vi "Video.vi"(8 "error in (no error)":errorcluster, 9 "title":string, 10 "id":string, 11 "Video in":refnum<class "Video.lvclass">) -> (0 "error out":errorcluster, 3 "Video out":refnum<class "Video.lvclass">)   [LabVIEW 2017, in "Video.lvclass"]
uses:
  Video.lvclass
  Video.lvclass/Video.ctl
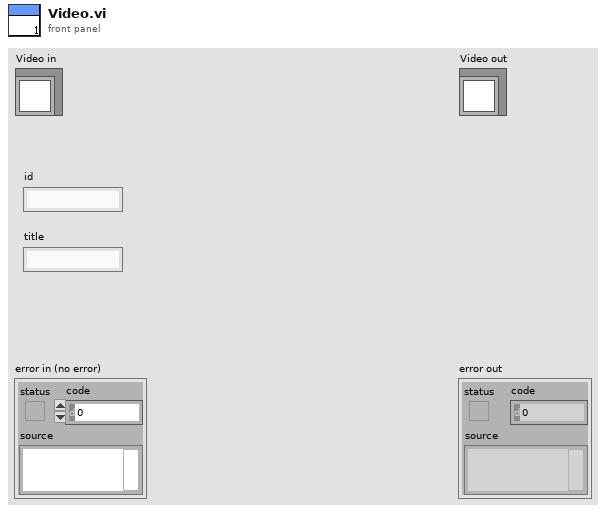
[diagram p1: front panel]
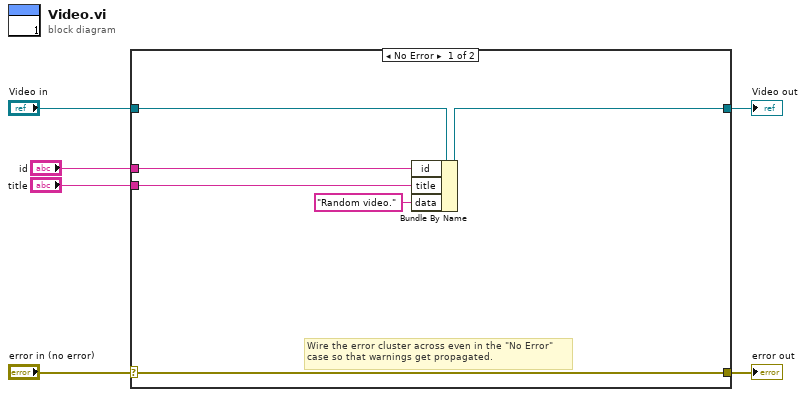
[diagram p0: block diagram]
diagram:
  n1 = case shown="No Error" "error in (no error)" {
    selector: "error in (no error)" -> [w11 w14]
    tunnel: [w11 w14] -> w5
    tunnel: [w10 w13] -> w3
    tunnel: "Video in" -> [w12 w13]
    tunnel: "id" -> [w9 _]
    tunnel: "title" -> [w8 _]
    frame No Error {
      # "Wire the error cluster across even in the \"No Error\"\ncase so that warnings get propagated."
      n2 = Bundle By Name(cluster=w12, "id"=w9, "title"=w8, "data"="Random video.") -> (w10:refnum<class "Video.lvclass">)
    }
    frame Error {
    }
  }
  "error out" <- w5
  "Video out" <- w3
